vi "vehicle_counting.vi"(0 "Array":T1(array[cluster]), 1 "Size":i32) -> (2 "Nom des couleurs":string[](array[string]), 3 "Occurences couleurs":dbl[](array[numeric]), 4 "Nombre de vehicules":dbl)   [LabVIEW 2024]
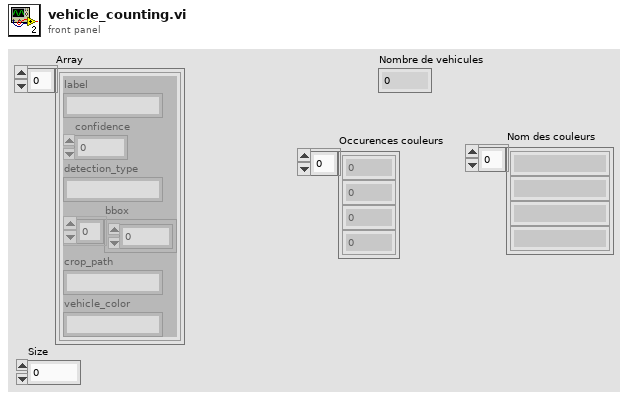
[diagram p1: front panel]
types:
  T1 = cluster{"label":string, "confidence":i32, "detection_type":string, "bbox":dbl[], "crop_path":string, "vehicle_color":string}[]
  T2 = cluster{"label":string, "confidence":i32, "detection_type":string, "bbox":dbl[], "crop_path":string, "vehicle_color":string}
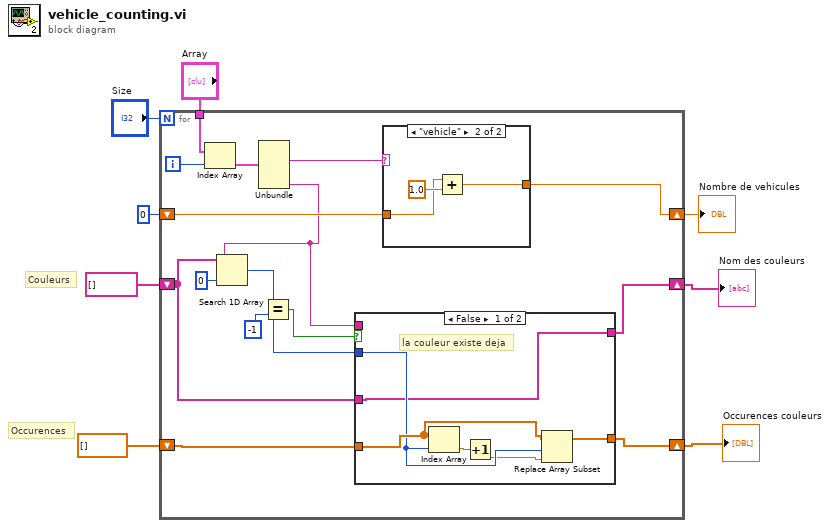
[diagram p0: block diagram]
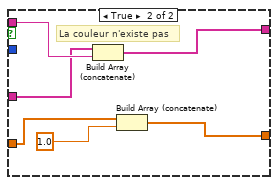
[diagram p2: hidden frame]
diagram:
  # "Occurences"
  # "Couleurs"
  n1 = for {
    N: "Size" -> [_]
    tunnel: "Array" -> [w22]
    shift-right: [w10] -> w5
    shift-left: 0 -> [w19]
    shift-right: [w11] -> w2
    shift-left: string[] [] ("Nom des couleurs 2") -> [w12]
    shift-right: [w14] -> w1
    shift-left: dbl[] [] ("Occurences 2") -> [w16]
    i -> [w23]
    n2 = Index Array(array=w22, index=w23) -> (element=w21:T2)
    n3 = Unbundle(w21) -> ("detection_type"=w20:string, "vehicle_color"=w13:string)  [unwired: 4 out]
    n4 = Search 1D Array(1D array=w12, element=w13, start index (0)=0) -> (index of element=w15:i32)
    n5 = Equal?(x=w15, y=-1) -> (x = y?=w17:bool)
    n6 = case shown="False" w17 {
      tunnel: w16 -> [w28 w31]
      tunnel: w15 -> [w27 _]
      tunnel: [w25 w30] -> w14
      tunnel: w13 -> [_ w35]
      tunnel: w12 -> [w24 w34]
      tunnel: [w24 w33] -> w11
      frame False {
        # "la couleur existe deja"
        n7 = Index Array(array=w28, index=w27) -> (element=w29:dbl)
        n8 = Increment(x=w29) -> (x+1=w26:dbl)
        n9 = Replace Array Subset(array=w28, new element=w26, index=w27) -> (w25:dbl[])
      }
      frame True {
        # "La couleur n'existe pas"
        n10 = Build Array (concatenate)(w34, w35) -> (w33:string[])
        n11 = Build Array (concatenate)(w31, 1.0 ("element")) -> (w30:dbl[])
      }
    }
    n12 = case shown="\"vehicle\"" w20 {
      tunnel: w19 -> [w36 w38]
      tunnel: [w36 w37] -> w10
      frame "False", Default {
      }
      frame "vehicle" {
        n13 = Add(x=w38, y=1.0) -> (x+y=w37:dbl)
      }
    }
  }
  "Nombre de vehicules" <- w5
  "Nom des couleurs" <- w2
  "Occurences couleurs" <- w1
